vi "Float64 Create.vi"(8 "error in (no error)":errorcluster, 11 "DBL in":dbl) -> (0 "error out":errorcluster, 3 "Float64 DVR out":refnum<data-value>)   [LabVIEW 2010, in "MDSplus.lvlib"]
uses:
  <vilib>/MDSplus/Library/MDSplus.lvlib
  <vilib>/MDSplus/Classes/Data_Class/Scalar_Class/Float64_Class/Float64.lvclass
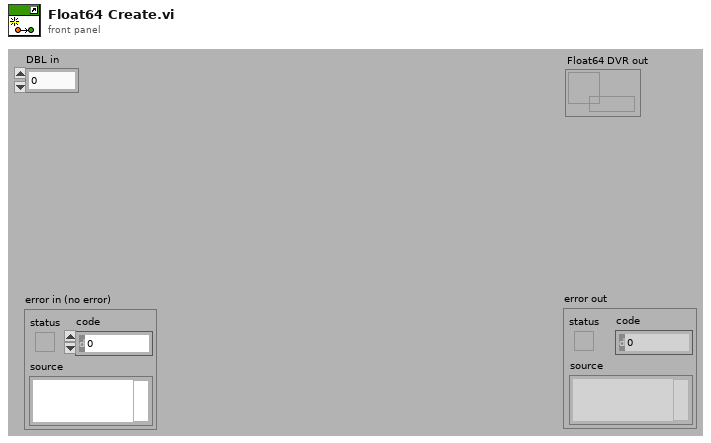
[diagram p1: front panel]
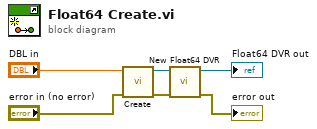
[diagram p0: block diagram]
diagram:
  n1 = call <vilib>:"Create.vi"("error in (no error)"="error in (no error)", "DBL in"="DBL in") -> ("error out"=w3:errorcluster, "Float64 out"=w4:refnum<class "Float64.lvclass">)  [unwired: 8 in]
  n2 = call <vilib>:"New Float64 DVR.vi"("error in (no error)"=w3, "Float64 in"=w4) -> ("error out"=→"error out":errorcluster, "Float64 DVR out"=→"Float64 DVR out":refnum<data-value>)  [unwired: 8 in]
